vi "oa_Draw Rotating Direction Indicator.vi"(5 "cartesian grid cosmetics":T1={"line color"=39168, "text color"=65280, "tick length(3)"=3, "crossing axes"=FALSE, "visible grid?"=TRUE}, 7 "picture \ndimensions (w,h)":cluster{"width":i16, "height":i16}, 8 "shaft rotating direction":u16(ring) items=["CCW", "CW"], 9 "plot type":u16(ring) items=["shaft centerline plot", "polar plot"], 11 "picture":picture) -> (3 "new picture":picture)   [LabVIEW 2017]
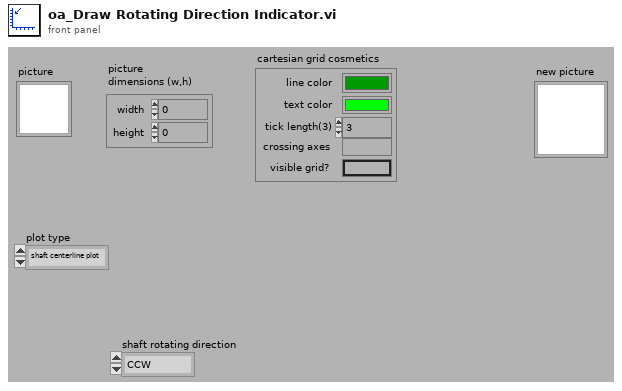
[diagram p1: front panel]
types:
  T1 = cluster{"line color":u32, "text color":u32, "tick length(3)":i16, "crossing axes":bool, "visible grid?":bool}
  T2 = cluster{"Width":u16, "Style":enum32{"Solid", "Dash", "Dot", "DashDot", "DashDotDot"}}
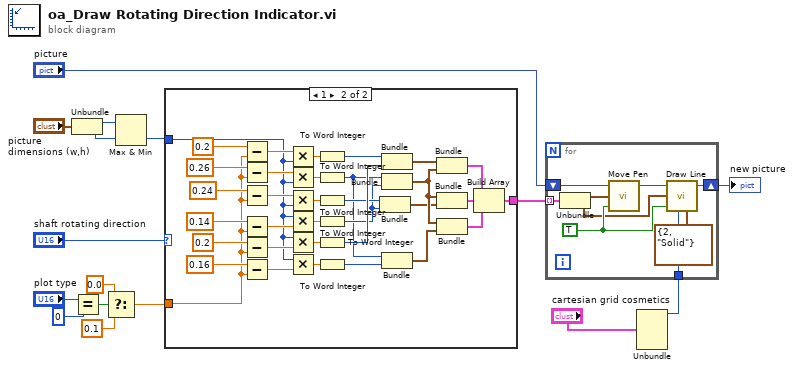
[diagram p0: block diagram]
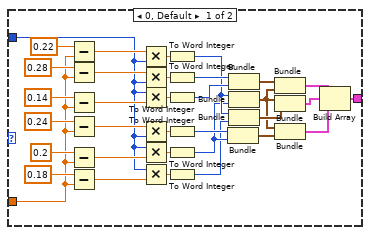
[diagram p2: hidden frame]
diagram:
  n1 = Unbundle("picture \ndimensions (w,h)") -> ("width"=w3:i16, "height"=w2:i16)
  n2 = Equal?(x="plot type", y=u16 0) -> (x = y?=w8:bool)
  n3 = Select(t=0.0 ("y"), s=w8, f=0.1 ("y")) -> (s? t:f=w5:dbl)
  n4 = Max & Min(x=w3, y=w2) -> (min(x,y)=w1:i16)  [unwired: 1 out]
  n5 = case shown="1" "shaft rotating direction" {
    tunnel: [w33 w66] -> w11
    tunnel: w5 -> [w18 w53]
    tunnel: w1 -> [w17 w52]
    frame 0, Default {
      n6 = Subtract(x=0.22, y=w18) -> (x-y=w26:dbl)
      n7 = Subtract(x=0.28, y=w18) -> (x-y=w25:dbl)
      n8 = Subtract(x=0.14, y=w18) -> (x-y=w21:dbl)
      n9 = Subtract(x=0.24, y=w18) -> (x-y=w23:dbl)
      n10 = Subtract(x=0.2, y=w18) -> (x-y=w20:dbl)
      n11 = Subtract(x=0.18, y=w18) -> (x-y=w19:dbl)
      n12 = Multiply(x=w26, y=w17) -> (x*y=w48:dbl)
      n13 = Multiply(x=w25, y=w17) -> (x*y=w47:dbl)
      n14 = Multiply(x=w17, y=w21) -> (x*y=w44:dbl)
      n15 = Multiply(x=w23, y=w17) -> (x*y=w46:dbl)
      n16 = Multiply(x=w17, y=w20) -> (x*y=w45:dbl)
      n17 = Multiply(x=w17, y=w19) -> (x*y=w27:dbl)
      n18 = To Word Integer(number=w48) -> (16bit integer=w34:i16)
      n19 = To Word Integer(number=w47) -> (16bit integer=w36:i16)
      n20 = To Word Integer(number=w44) -> (16bit integer=w35:i16)
      n21 = To Word Integer(number=w46) -> (16bit integer=w31:i16)
      n22 = To Word Integer(number=w45) -> (16bit integer=w30:i16)
      n23 = To Word Integer(number=w27) -> (16bit integer=w29:i16)
      n24 = Bundle(w31, w30) -> (w40:cluster{i16, i16})  [unwired: 1 in]
      n25 = Bundle(w36, w35) -> (w43:cluster{i16, i16})  [unwired: 1 in]
      n26 = Bundle(w34, w30) -> (w41:cluster{i16, i16})  [unwired: 1 in]
      n27 = Bundle(w34, w29) -> (w42:cluster{i16, i16})  [unwired: 1 in]
      n28 = Bundle(w43, w41) -> (w39:cluster{cluster{i16, i16}, cluster{i16, i16}})  [unwired: 1 in]
      n29 = Bundle(w41, w42) -> (w38:cluster{cluster{i16, i16}, cluster{i16, i16}})  [unwired: 1 in]
      n30 = Bundle(w41, w40) -> (w37:cluster{cluster{i16, i16}, cluster{i16, i16}})  [unwired: 1 in]
      n31 = Build Array(w39, w38, w37) -> (w33:cluster{cluster{i16, i16}, cluster{i16, i16}}[])
    }
    frame 1 {
      n32 = Subtract(x=0.2, y=w53) -> (x-y=w60:dbl)
      n33 = Subtract(x=0.26, y=w53) -> (x-y=w58:dbl)
      n34 = Subtract(x=0.24, y=w53) -> (x-y=w57:dbl)
      n35 = Subtract(x=0.14, y=w53) -> (x-y=w56:dbl)
      n36 = Subtract(x=0.2, y=w53) -> (x-y=w55:dbl)
      n37 = Subtract(x=0.16, y=w53) -> (x-y=w54:dbl)
      n38 = Multiply(x=w60, y=w52) -> (x*y=w81:dbl)
      n39 = Multiply(x=w58, y=w52) -> (x*y=w80:dbl)
      n40 = Multiply(x=w57, y=w52) -> (x*y=w79:dbl)
      n41 = Multiply(x=w52, y=w56) -> (x*y=w77:dbl)
      n42 = Multiply(x=w52, y=w55) -> (x*y=w78:dbl)
      n43 = Multiply(x=w52, y=w54) -> (x*y=w76:dbl)
      n44 = To Word Integer(number=w81) -> (16bit integer=w63:i16)
      n45 = To Word Integer(number=w80) -> (16bit integer=w51:i16)
      n46 = To Word Integer(number=w79) -> (16bit integer=w70:i16)
      n47 = To Word Integer(number=w77) -> (16bit integer=w69:i16)
      n48 = To Word Integer(number=w78) -> (16bit integer=w75:i16)
      n49 = To Word Integer(number=w76) -> (16bit integer=w74:i16)
      n50 = Bundle(w70, w69) -> (w68:cluster{i16, i16})  [unwired: 1 in]
      n51 = Bundle(w63, w75) -> (w73:cluster{i16, i16})  [unwired: 1 in]
      n52 = Bundle(w51, w69) -> (w71:cluster{i16, i16})  [unwired: 1 in]
      n53 = Bundle(w51, w74) -> (w72:cluster{i16, i16})  [unwired: 1 in]
      n54 = Bundle(w73, w71) -> (w67:cluster{cluster{i16, i16}, cluster{i16, i16}})  [unwired: 1 in]
      n55 = Bundle(w71, w68) -> (w62:cluster{cluster{i16, i16}, cluster{i16, i16}})  [unwired: 1 in]
      n56 = Bundle(w71, w72) -> (w61:cluster{cluster{i16, i16}, cluster{i16, i16}})  [unwired: 1 in]
      n57 = Build Array(w67, w62, w61) -> (w66:cluster{cluster{i16, i16}, cluster{i16, i16}}[])
    }
  }
  n58 = Unbundle("cartesian grid cosmetics") -> ("line color"=w13:u32)  [unwired: 4 out]
  n59 = for {
    shift-right: [w93] -> w15
    shift-left: "picture" -> [w91]
    tunnel: w13 -> [w92]
    tunnel: w11 -> [w87] mode=indexing
    w89 = TRUE ("absolute coordinates?(T)")
    n60 = Unbundle(w87) -> (w86:cluster{i16, i16}, w85:cluster{i16, i16})
    n61 = call <vilib>:"Move Pen.vi"("absolute coordinates?(T)"=w89, "new position"=w86, "picture"=w91) -> ("new picture"=w90:picture)  [unwired: 2 in]
    n62 = call <vilib>:"Draw Line.vi"("picture"=w90, "end point"=w85, "absolute coordinates?(T)"=w89, "color(black)"=w92, "pen"=T2 {"Width"=2, "Style"=enum."Solid"}) -> ("new picture"=w93:picture)  [unwired: 4 in]
  }
  "new picture" <- w15
